vi "laba4.vi"() -> ()   [LabVIEW 2018]
panel:
  in  "Амплитуда":dbl(knob) scale=0.0..10.0
  in  "stop":bool
  out "Sweep Chart":cluster{dbl, dbl}(graph)
  out "Scope Chart":cluster{dbl, dbl}(graph)
  out "Strip Chart":cluster{dbl, dbl}(graph)
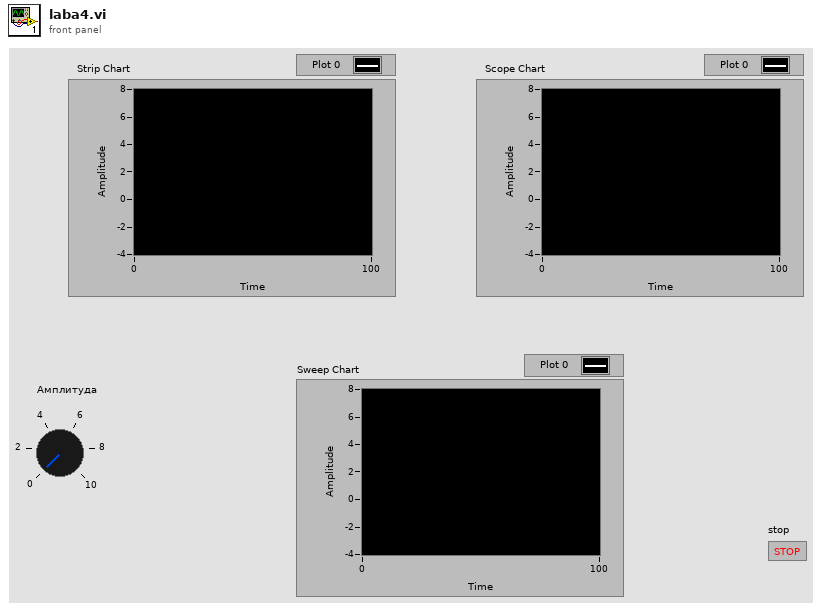
[diagram p1: front panel]
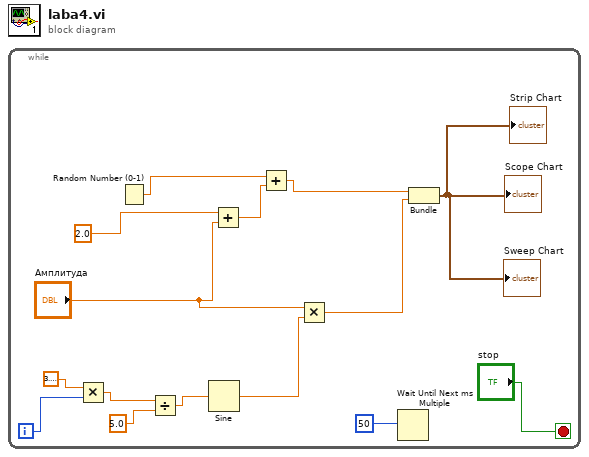
[diagram p0: block diagram]
diagram:
  n1 = while {
    i -> [w9]
    stop <- "stop" stop-if-true
    n2 = Multiply(x=3.141592653589793, y=w9) -> (x*y=w7:dbl)
    n3 = Random Number (0-1)() -> (number: 0 to 1=w13:dbl)
    n4 = Divide(x=w7, y=5.0) -> (x/y=w5:dbl)
    n5 = Sine(x=w5) -> (sin(x)=w3:dbl)
    n6 = Add(x=2.0, y="Амплитуда") -> (x+y=w12:dbl)
    n7 = Add(x=w13, y=w12) -> (x+y=w11:dbl)
    n8 = Multiply(x="Амплитуда", y=w3) -> (x*y=w2:dbl)
    n9 = Wait Until Next ms Multiple(millisecond multiple=50) -> ()  [unwired: 1 out]
    n10 = Bundle(w11, w2) -> (→"Strip Chart" →"Scope Chart" →"Sweep Chart":cluster{dbl, dbl})  [unwired: 1 in]
  }
